vi "Set Scale Name.vi"(8 "error in (no error)":errorcluster, 9 "references":T1, 10 "name":string, 11 "index":i32) -> (0 "error out":errorcluster)   [LabVIEW 2015, in "Scaling editor node.lvclass"]
uses:
  Scaling editor node.lvclass
  <vilib>/NI/DCAF Table API/Table Manager/object ref.ctl
  <vilib>/NI/Tag Bus Data Framework/Configuration Editor/Classes/Engine Parent/Engine Parent Editor Node.lvclass
  <vilib>/NI/Tag Bus Data Framework/Configuration Editor/Classes/Module editor node/module editor node.lvclass
  module/configuration/Scaling configuration.lvclass
  <vilib>/NI/DCAF Table API/Table Manager/Table Manager.lvclass
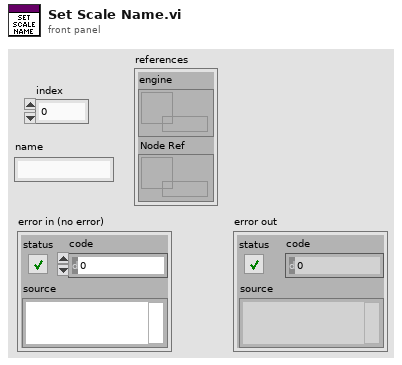
[diagram p1: front panel]
types:
  T1 = typedef "Table Manager.lvlib/Table Manager.lvclass/object ref.ctl" = cluster{"engine":refnum<data-value>, "Node Ref":refnum<data-value>}
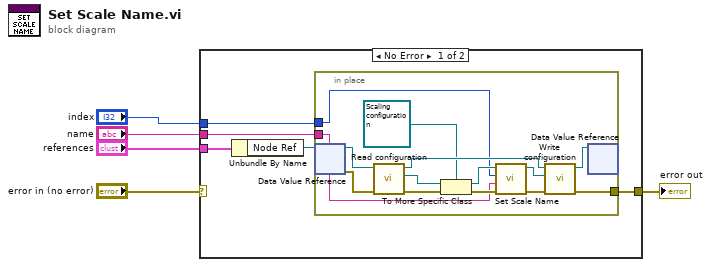
[diagram p0: block diagram]
diagram:
  n1 = case shown="No Error" "error in (no error)" {
    selector: "error in (no error)" -> [_ w25]
    tunnel: [w10 w25] -> w3
    tunnel: "index" -> [w8 _]
    tunnel: "references" -> [w7 _]
    tunnel: "name" -> [w6 _]
    frame No Error {
      n2 = Unbundle By Name(w7) -> ("Node Ref"=w9:refnum<data-value>)
      n3 = in-place {
        in-place-border: [w20] -> w10
        in-place-border: w8 -> [w14]
        in-place-border: w6 -> [w13]
        n4 = in-place-dvr #1(w9) -> (w23:refnum<class "module editor node.lvclass">, w19:errorcluster)
        n5 = call-dynamic "Read configuration.vi"("error in"=w19, "NISE_CEF_serializable node in"=w23) -> ("error out"=w18:errorcluster, "configuration"=w22:refnum<class "NISE_CEF_serializable configuration.lvclass">, "NISE_CEF_serializable node out"=w24:refnum<class "module editor node.lvclass">)  [unwired: 7 in]
        n6 = To More Specific Class(target class=refnum<class "Scaling configuration.lvclass"> refnum ("Scaling configuration"), reference=w22, error in=w18) -> (specific class reference=w15:refnum<class "Scaling configuration.lvclass">, error out=w16:errorcluster)
        n7 = call "Set Scale Name.vi"("error in (no error)"=w16, "name"=w13, "index"=w14, "Scaling configuration in"=w15) -> ("error out"=w11:errorcluster, "Scaling configuration out"=w12:refnum<class "Scaling configuration.lvclass">)  [unwired: 6 in]
        n8 = call-dynamic "Write configuration.vi"("error in"=w11, "configuration"=w12, "NISE_CEF_serializable node in"=w24) -> ("error out"=w20:errorcluster, "NISE_CEF_serializable node out"=w21:refnum<class "module editor node.lvclass">)  [unwired: 7 in]
        n9 = in-place-dvr #1(w21) -> ()  [unwired: 2 out]
      }
    }
    frame Error {
    }
  }
  "error out" <- w3
